vi "CBR_GetInstance.vi"(3 "App.ContextName":string="Main Application Instance") -> (1 "Application out":refnum<vi>)   [LabVIEW 2012]
panel:
  out "Instances":string[](array[string])
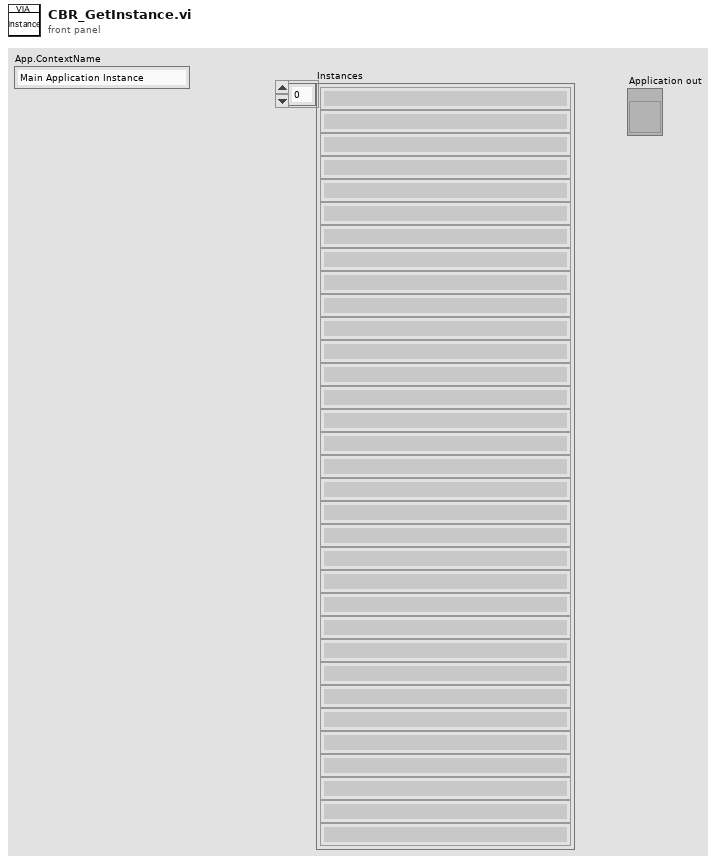
[diagram p1: front panel]
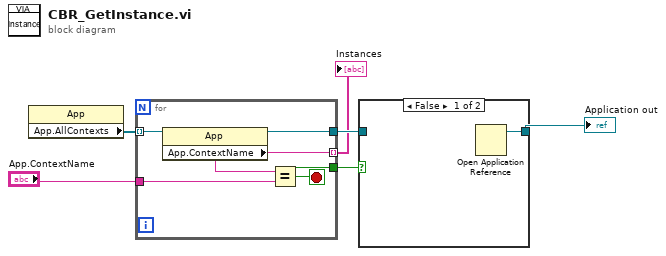
[diagram p0: block diagram]
diagram:
  n1 = property class="App"() -> ("App.AllContexts"=w1:refnum<vi>[])  [unwired: 2 in, 2 out]
  n2 = for {
    tunnel: w1 -> [w11] mode=indexing
    tunnel: [w10] -> w4
    tunnel: [w9] -> w2 mode=indexing
    tunnel: "App.ContextName" -> [w8]
    tunnel: [w7] -> w3
    stop <- w7 stop-if-true
    n3 = property class="App"(reference=w11) -> (reference out=w10:refnum<vi>, "App.ContextName"=w9:string)  [unwired: 1 in, 1 out]
    n4 = Equal?(x=w9, y=w8) -> (x = y?=w7:bool)
  }
  "Instances" <- w2
  n5 = case shown="False" w3 {
    tunnel: [w12 w13] -> w6
    tunnel: w4 -> [_ w13]
    frame False {
      n6 = Open Application Reference() -> (3:w12:refnum<vi>)  [unwired: 4 in, 1 out]
    }
    frame True {
    }
  }
  "Application out" <- w6
